vi "Constant_Speed_Final.vi"() -> ()   [LabVIEW 2024]
uses:
  <vilib>/Analysis/baseanly.llb/Real A x B.vi
  <vilib>/Analysis/baseanly.llb/Real Inverse Matrix.vi
  <vilib>/Analysis/NI_AALBase.lvlib
panel:
  in  "VISA Refnum in":refnum<visa-resource-name>
  out "end (2D)":cluster{"x":dbl, "y":dbl}
  in  "picture in":picture
  out "end effector":cluster{"X":dbl, "Y":dbl}={"X"=61.080020351084045, "Y"=-1.710100716628343}
  in  "geometry?":bool
  in  "arms":T1(array[cluster])=[{"Translation"={"X"=0.0, "Y"=0.0, "Z"=0.0}, "Axis"=enum."z", "Angle (degrees)"=20.0}, {"Translation"={"X"=30.0, "Y"=0.0, "Z"=0.0}, "Axis"=enum."z", "Angle (degrees)"=-40.0}, {"Translation"={"X"=35.0, "Y"=0.0, "Z"=0.0}, "Axis"=enum."z", "Angle (degrees)"=0.0}] {"Angle (degrees)" scale=0.0..180.0}
  out "2D Picture":picture
  out "q2":dbl
  out "q1":dbl
  in  "stop":bool
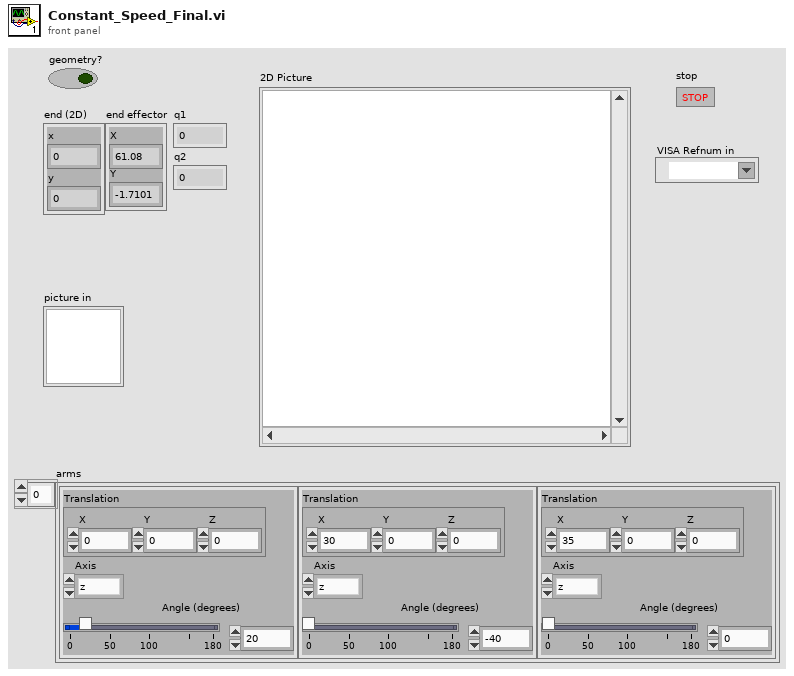
[diagram p1: front panel]
types:
  T1 = cluster{"Translation":cluster{"X":dbl, "Y":dbl, "Z":dbl}, "Axis":enum16{"x", "y", "z"}, "Angle (degrees)":dbl}[]
  T2 = typedef "NI_Matrix.lvlib/RealMatrix.ctl" = dbl[][]
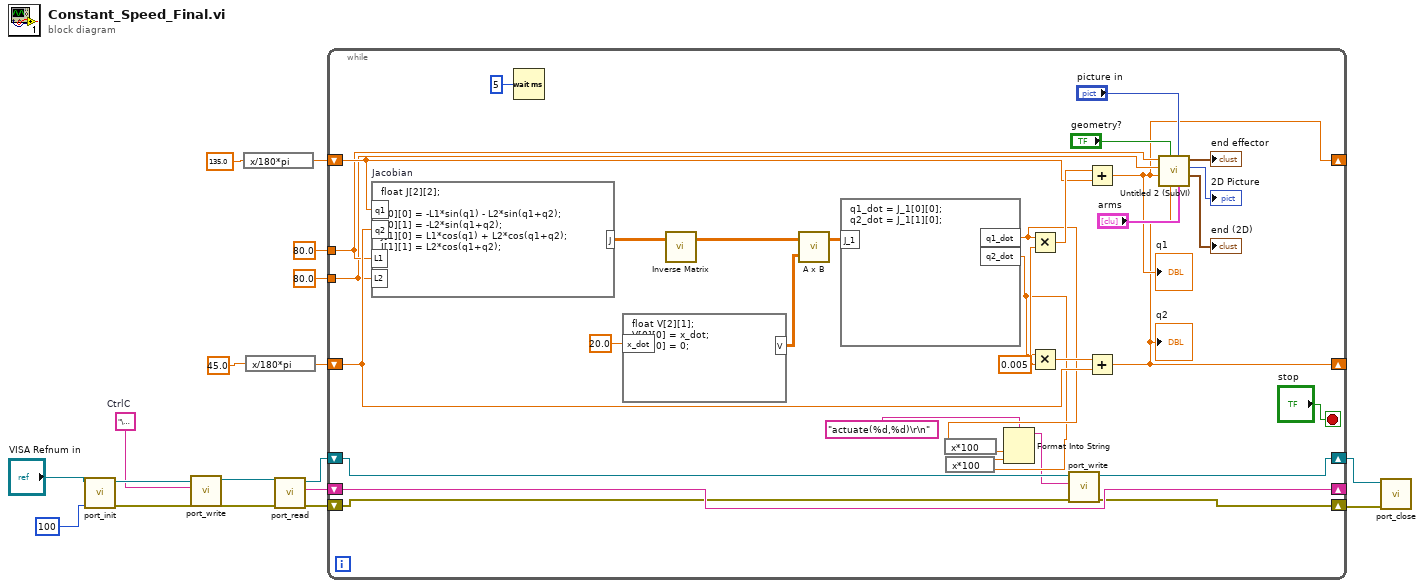
[diagram p0: block diagram]
diagram:
  w8 = "\u0003"  # CtrlC
  n1 = call <userlib>:"port_init.vi"("Timeout (ms)"=u32 100, "VISA Refnum in"="VISA Refnum in") -> ("error out"=w10:errorcluster, "VISA Refnum out"=w9:refnum<visa-resource-name>)  [unwired: 8 in]
  n2 = call <userlib>:"port_write.vi"("error in (no error)"=w10, "write buffer"=w8, "VISA Refnum in"=w9) -> ("error out"=w1:errorcluster, "VISA Refnum out"=w2:refnum<visa-resource-name>)  [unwired: 7 in]
  n3 = expression code="x/180*pi"(135.0) -> (w14:dbl)
  n4 = expression code="x/180*pi"(45.0) -> (w13:dbl)
  n5 = call <userlib>:"port_read.vi"("error in (no error)"=w1, "VISA Refnum in"=w2) -> ("error out"=w5:errorcluster, "reply"=w6:string, "VISA Refnum out"=w7:refnum<visa-resource-name>)  [unwired: 7 in]
  n6 = while {
    shift-right: [w31] -> _
    shift-left: w14 -> [w41]
    shift-right: [w30] -> _
    shift-left: w13 -> [w40]
    tunnel: 80.0 -> [w33]
    tunnel: 80.0 -> [w32]
    shift-right: [w27] -> w3
    shift-left: w7 -> [w28]
    shift-right: [w29] -> _
    shift-left: w6 -> [w29]
    shift-right: [w25] -> w4
    shift-left: w5 -> [w26]
    stop <- "stop" stop-if-true
    w44 = 0.005
    n7 = formula code="float J[2][2];\n\nJ[0][0] = -L1*sin(q1) - L2*sin(q1+q2);\nJ[0][1] = -L2*sin(q1+q2);\nJ[1][0] = L1*cos(q1) + L2*cos(q1+q2);\nJ[1][1] = L2*cos(q1+q2);" "Jacobian"("q1"=w41, "q2"=w40, "L1"=w33, "L2"=w32) -> ("J"=w51:dbl[][])
    n8 = Wait (ms)(milliseconds to wait=u32 5) -> ()  [unwired: 1 out]
    n9 = formula code="float V[2][1];\nV[0][0] = x_dot;\nV[1][0] = 0;"("x_dot"=20.0 ("input variable")) -> ("V"=w48:dbl[][])
    n10 = call-poly <vilib>:"Inverse Matrix.vi"("Input Matrix"=w51) -> ("Inverse Matrix"=w50:T2)  [unwired: 1 in, 1 out]
    n11 = call-poly <vilib>:"A x B.vi"("B"=w48, "A"=w50) -> ("A x B"=w46:T2)  [unwired: 1 out]
    n12 = formula code="q1_dot = J_1[0][0];\nq2_dot = J_1[1][0];"("J_1"=w46) -> ("q1_dot"=w24:dbl, "q2_dot"=w23:dbl)
    n13 = expression code="x*100"(w24) -> (w20:dbl)
    n14 = expression code="x*100"(w23) -> (w19:dbl)
    n15 = Format Into String(format string="actuate(%d,%d)\r\n", w20, w19) -> (resulting string=w21:string)  [unwired: 2 in, 1 out]
    n16 = Multiply(x=w24, y=w44) -> (x*y=w43:dbl)
    n17 = Multiply(x=w23, y=w44) -> (x*y=w42:dbl)
    n18 = call <userlib>:"port_write.vi"("error in (no error)"=w26, "write buffer"=w21, "VISA Refnum in"=w28) -> ("error out"=w25:errorcluster, "VISA Refnum out"=w27:refnum<visa-resource-name>)  [unwired: 7 in]
    n19 = Add(x=w43, y=w41) -> (x+y=w31:dbl)
    "q1" <- w31
    n20 = Add(x=w42, y=w40) -> (x+y=w30:dbl)
    "q2" <- w30
    n21 = call "Untitled 2 (SubVI).vi"("arms"="arms", "picture in"="picture in", "input variable 3"=w30, "geometry?"="geometry?", "input variable"=w31, "input variable 2"=w32, "input variable 4"=w33) -> ("end (2D)"=→"end (2D)":cluster{"x":dbl, "y":dbl}, "2D Picture"=→"2D Picture":picture, "end effector"=→"end effector":cluster{"X":dbl, "Y":dbl})  [unwired: 2 in]
  }
  n22 = call <userlib>:"port_close.vi"("error in (no error)"=w4, "VISA Refnum in"=w3) -> ()  [unwired: 10 in]
